vi "Write VISA resource name.vi"(8 "error in (no error)":errorcluster, 10 "VISA resource name":refnum<visa-resource-name>, 11 "Eurotherm 3200 PID Controller in":refnum<class "Eurotherm 3200 PID Controller.lvclass">) -> (0 "error out":errorcluster, 3 "Eurotherm 3200 PID Controller out":refnum<class "Eurotherm 3200 PID Controller.lvclass">)   [LabVIEW 2011, in "Eurotherm 3200 PID Controller.lvclass"]
uses:
  Eurotherm 3200 PID Controller.lvclass
  Eurotherm 3200 PID Controller.lvclass/Eurotherm 3200 PID Controller.ctl
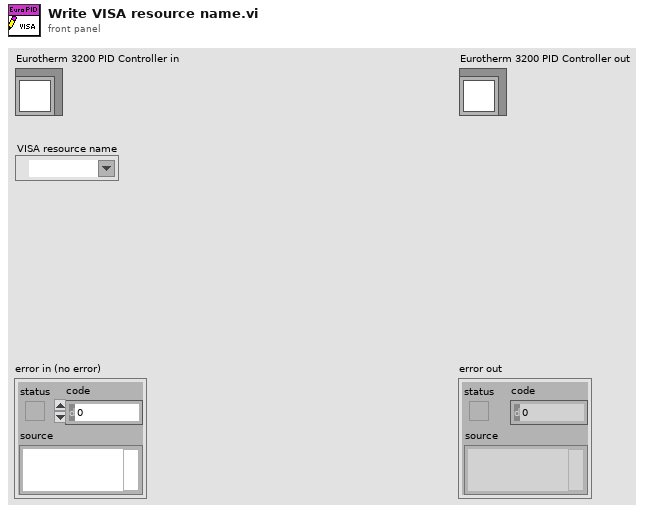
[diagram p1: front panel]
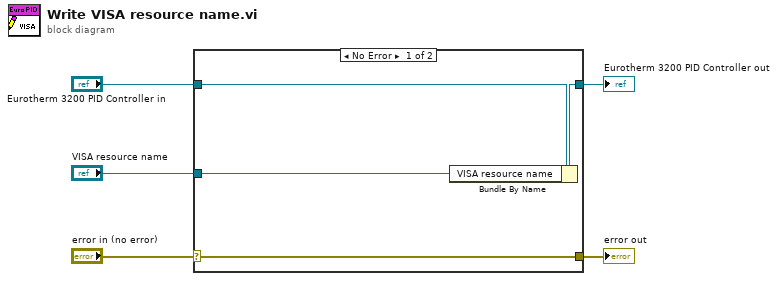
[diagram p0: block diagram]
diagram:
  n1 = case shown="No Error" "error in (no error)" {
    selector: "error in (no error)" -> [w9 w10]
    tunnel: [w9 w10] -> w4
    tunnel: [w7 w11] -> w2
    tunnel: "Eurotherm 3200 PID Controller in" -> [w8 w11]
    tunnel: "VISA resource name" -> [w6 _]
    frame No Error {
      n2 = Bundle By Name(cluster=w8, "VISA resource name"=w6) -> (w7:refnum<class "Eurotherm 3200 PID Controller.lvclass">)
    }
    frame Error {
    }
  }
  "error out" <- w4
  "Eurotherm 3200 PID Controller out" <- w2
